vi "MCCMSG Get Meter Value.vi"(7 "pnError":i32, 8 "error in (no error)":errorcluster, 9 "uMeterID":u32, 10 "pdValue":dbl, 11 "hMCCmsg":i32) -> (0 "error out":errorcluster, 2 "pdValue out":dbl, 3 "function return":i32, 5 "pnError out":i32)   [LabVIEW 2012, in "MultiClamp 700B Controls.lvlib" / "AxMultiClampMsg.lvlib"]
doc: "AXMCCMSG BOOL WINAPI MCCMSG_GetMeterValue(HMCCMSG hMCCmsg, double *pdValue, UINT uMeterID, int *pnError);"
uses:
  AxMultiClampMsg.lvlib
  AxMultiClampMsg.dll
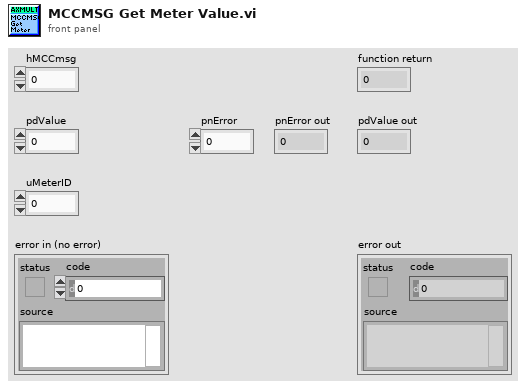
[diagram p1: front panel]
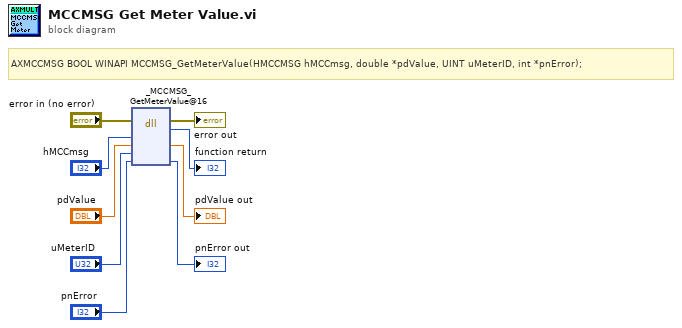
[diagram p0: block diagram]
diagram:
  # "AXMCCMSG BOOL WINAPI MCCMSG_GetMeterValue(HMCCMSG hMCCmsg, double *pdValue, UINT uMeterID, int *pnError);"
  n1 = dll-call lib="C:/Users/LAA12/Desktop/Rita/Multiclamp 700B VIs/AxMultiClampMsg/AxMultiClampMsg.*" fn="_MCCMSG_GetMeterValue@16"(error in="error in (no error)", "hMCCmsg"="hMCCmsg", "pdValue"="pdValue", "uMeterID"="uMeterID", "pnError"="pnError") -> (error out=→"error out":errorcluster, →"function return":i32, "pdValue"=→"pdValue out":dbl, "pnError"=→"pnError out":i32)  [unwired: 4 in, 1 out]
